vi "Main Server.vi"(11 "tCRD in":refnum<class "Aircraft OPCCRD.lvclass">) -> (0 "error out":errorcluster)   [LabVIEW 2015]
uses:
  CRD/Aircraft OPCCRD.lvclass
  Reusable/Instrument/state.ctl
  Reusable/Session Log/System Log.lvclass
  CRD/Data/tCRD Data.lvclass
  Reusable/Session Log/System Log.lvclass/System Log.ctl
  Reusable/Instrument/Instrument.lvclass/Instrument.ctl
  Reusable/Session Log/Accessors/Write Main Path.vi
  Reusable/Instrument/Write Log Session.vi
  Reusable/CRDS/Main/Write Data.vi
  Reusable/Instrument/Instrument.lvclass
  <userlib>/_Session Fwk/Session - Root.lvclass
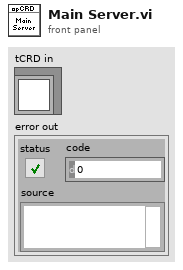
[diagram p1: front panel]
types:
  T1 = typedef "Instrument.lvclass/state.ctl" = enum8{"Configure", "Acquire", "Wait", "Quit", "Handle Error", "NOOP"}
  T2 = typedef "Session - Root.lvclass/Session Handle.ctl" = refnum<data-value>
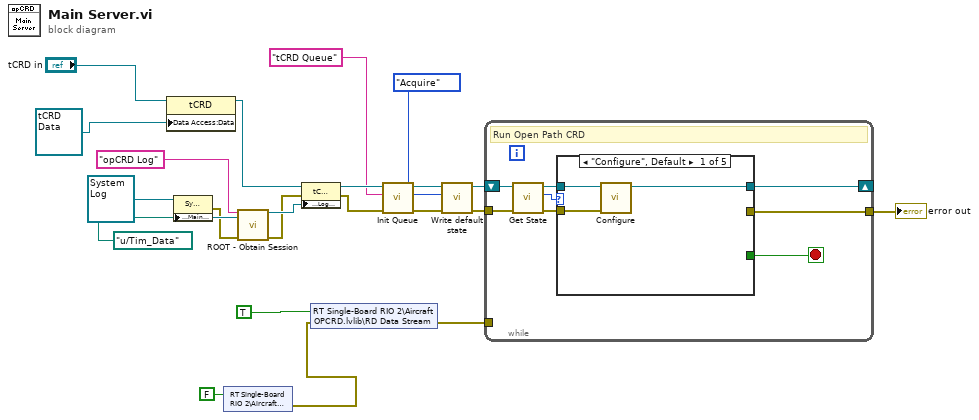
[diagram p0: block diagram]
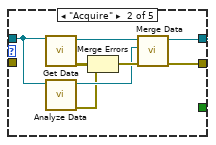
[diagram p2: hidden frame]
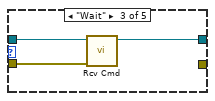
[diagram p3: hidden frame]
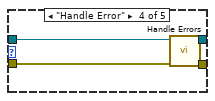
[diagram p4: hidden frame]
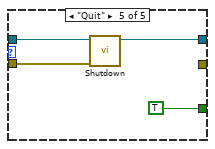
[diagram p5: hidden frame]
diagram:
  n1 = property class="tCRD"(reference="tCRD in", "Data Access:Data"=refnum<class "tCRD Data.lvclass"> refnum ("tCRD Data")) -> (reference out=w4:refnum<class "Aircraft OPCCRD.lvclass">)  [unwired: 1 in, 1 out]
  n2 = property class="Sys Log"(reference=refnum<class "System Log.lvclass"> refnum ("Sys Log"), "Accessors:Main Path"=path "u:/Tim_Data" ("RD Data Path")) -> (reference out=w14:refnum<class "System Log.lvclass">, error out=w13:errorcluster)  [unwired: 1 in]
  n3 = shared-variable "RT Single-Board RIO 2\\Aircraft OPCRD.lvlib\\Stop"(FALSE ("Stop")) -> (error out=w2:errorcluster)  [unwired: 1 in]
  n4 = call <userlib>:"ROOT - Obtain Session.vi"("Session Name ()"="opCRD Log", "OBJ - Session"=w14, "error in (no error)"=w13) -> ("Session Handle"=w11:T2, "error out"=w10:errorcluster)  [unwired: 10 in, 1 out]
  n5 = property class="tCRD"(reference=w4, error in=w10, "Accessors:Log Session"=w11) -> (reference out=w22:refnum<class "Aircraft OPCCRD.lvclass">, error out=w6:errorcluster)
  n6 = shared-variable "RT Single-Board RIO 2\\Aircraft OPCRD.lvlib\\RD Data Stream"(TRUE ("RD Data Stream"), error in=w2) -> (error out=w7:errorcluster)
  n7 = call "Init Queue.vi"("error in"=w6, "queue_name"="tCRD Queue", "Instrument in"=w22) -> ("error out"=w21:errorcluster, "Instrument out"=w20:refnum<class "Aircraft OPCCRD.lvclass">)  [unwired: 7 in]
  n8 = call "Write default state.vi"("error in (no error)"=w21, "instr state"=state."Acquire", "Instrument in"=w20) -> ("error out"=w23:errorcluster, "Instrument out"=w19:refnum<class "Aircraft OPCCRD.lvclass">)  [unwired: 7 in]
  n9 = while "Acquisition" {
    tunnel: w23 -> [w31]
    shift-right: [w28] -> _
    shift-left: w19 -> [w30]
    tunnel: [w27] -> w9
    tunnel: w7 -> [_]
    stop <- w29 stop-if-true
    # "Run Open Path CRD"
    n10 = call "Get State.vi"("error in"=w31, "Instrument in"=w30) -> ("error out"=w24:errorcluster, "default state"=w26:T1, "Instrument out"=w25:refnum<class "Aircraft OPCCRD.lvclass">)  [unwired: 7 in]
    n11 = case shown="\"Configure\", Default" w26 {
      tunnel: w25 -> [w34 w41 w44 w48 w51]
      tunnel: w24 -> [w33 _ w43 w47 w50]
      tunnel: [_ _ _ _ TRUE] -> w29
      tunnel: [w32 w42 w45 w46 w49] -> w28
      tunnel: [_ w40 _ _ _] -> w27
      frame "Configure", Default {
        n12 = call-dynamic "Configure.vi"("error in"=w33, "tCRD in"=w34) -> ("tCRD out"=w32:refnum<class "Aircraft OPCCRD.lvclass">)  [unwired: 8 in, 1 out]
      }
      frame "Acquire" {
        n13 = call-dynamic "Get Data.vi"("tCRD in"=w41) -> ("error out"=w36:errorcluster, "tCRD out"=w39:refnum<class "Aircraft OPCCRD.lvclass">)  [unwired: 9 in]
        n14 = call-dynamic "Analyze Data.vi"("tCRD in"=w41) -> ("error out"=w35:errorcluster, "tCRD out"=w37:refnum<class "Aircraft OPCCRD.lvclass">)  [unwired: 9 in]
        n15 = Merge Errors(w36, w35) -> (w38:errorcluster)
        n16 = call-dynamic "Merge Data.vi"("error in"=w38, "Analyzed"=w37, "Acquired"=w39) -> ("error out"=w40:errorcluster, "tCRD out"=w42:refnum<class "Aircraft OPCCRD.lvclass">)  [unwired: 7 in]
      }
      frame "Wait" {
        n17 = call-dynamic "Rcv Cmd.vi"("error in"=w43, "tCRD in"=w44) -> ("tCRD out"=w45:refnum<class "Aircraft OPCCRD.lvclass">)  [unwired: 8 in, 1 out]
      }
      frame "Handle Error" {
        n18 = call-dynamic "Handle Errors.vi"("error in"=w47, "tCRD in"=w48) -> ("tCRD out"=w46:refnum<class "Aircraft OPCCRD.lvclass">)  [unwired: 7 in, 2 out]
      }
      frame "Quit" {
        n19 = call-dynamic "Shutdown.vi"("error in"=w50, "tCRD in"=w51) -> ("tCRD out"=w49:refnum<class "Aircraft OPCCRD.lvclass">)  [unwired: 8 in, 1 out]
      }
    }
  }
  "error out" <- w9
